vi "ExitLabVIEW.vi"(11 "ErrorIn":errorcluster) -> (15 "ErrorOut":errorcluster)   [LabVIEW 2018]
doc: "Check to see if this is a Run Time application and if so, exit LabVIEW. This can be handy: when the default settings are in place, LabVIEW cleans up resources upon exit, such as closing GPIB connections and releasing memory.\n\nChecking for Run Time System status (in other words, checking if this is an EXE) is useful during development so that we don't exit LabVIEW when running this VI in development mode.\n\nCopyright © 2019 Epimedia, Inc. All Rights Reserved.\n\nThe Epimedia Application Library is Copyright © 2009-2019 Epimedia, Inc. \nAll Rights Reserved. Used under license."
panel:
  # "Copyright © 2019 Epimedia, Inc. All Rights Reserved.\n\nThe Epimedia Application Library is Copyright © 2009-2019 Epimedia, Inc. \nAll Rights Reserved. Used under license."
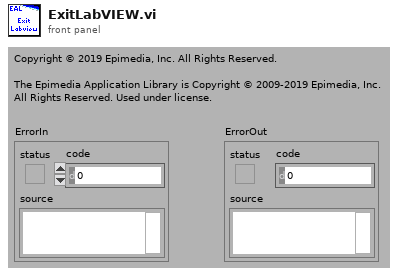
[diagram p1: front panel]
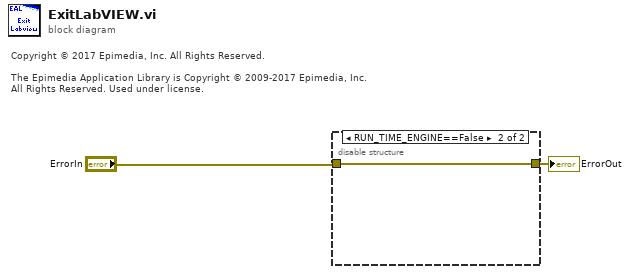
[diagram p0: block diagram]
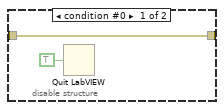
[diagram p2: hidden frame]
diagram:
  # "Copyright © 2017 Epimedia, Inc. All Rights Reserved.\n\nThe Epimedia Application Library is Copyright © 2009-2017 Epimedia, Inc. \nAll Rights Reserved. Used under license."
  n1 = disable-structure shown="RUN_TIME_ENGINE==False" {
    disable-tunnel: [w3 w5] -> w2
    disable-tunnel: "ErrorIn" -> [w3 w5]
    frame condition #0 {
      n2 = Quit LabVIEW(quit? (T)=TRUE) -> ()
    }
    frame condition #1 (active) {
    }
  }
  "ErrorOut" <- w2
